vi "Get Parallel Sinks.vi"(8 "error in (no error)":errorcluster, 11 "Application Log in":refnum<class "Application Log.lvclass">) -> (0 "error out":errorcluster, 3 "Application Log out":refnum<class "Application Log.lvclass">, 5 "Parallel Sinks":bool)   [LabVIEW 2016, in "Stream Log.lvlib" / "Application Log.lvclass"]
doc: "--\nCopyright © 2017 Composed SystemsI All rights reserved.\n\nAuthor: Jon McBee <jon.mcbee@composed.io>\n\nThis library is provided \"AS IS\" ,WITHOUT WARRANTIES OR\nCONDITIONS OF ANY KIND, either express or implied.\n\nComposed Systems -- composed.io\n\nStream 0.0.1.1\nJon McBee - Composed Systems\nCopyright (c) 2017, Composed Systems"
uses:
  <userlib>/Composed Systems/Stream/Log/Application Log/Application Log.lvclass
  <userlib>/Composed Systems/Stream/Log/Application Log/Application Log.lvclass/Application Log.ctl
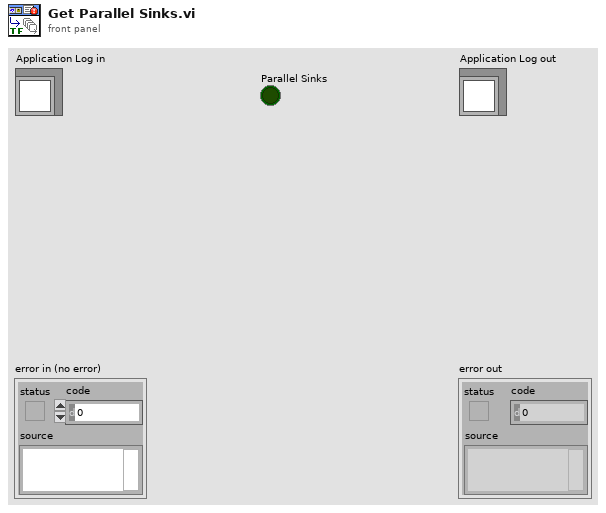
[diagram p1: front panel]
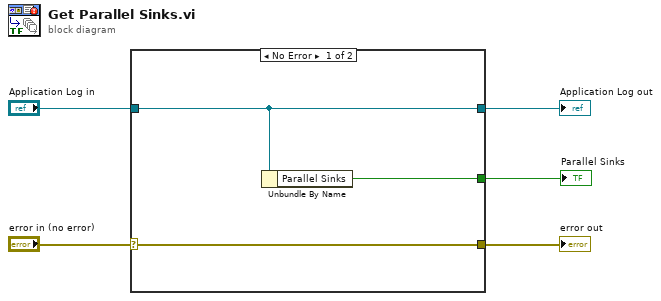
[diagram p0: block diagram]
diagram:
  n1 = case shown="No Error" "error in (no error)" {
    selector: "error in (no error)" -> [w8 w10]
    tunnel: [w8 w10] -> w4
    tunnel: [w7 w9] -> w2
    tunnel: "Application Log in" -> [w7 w9]
    tunnel: [w6 _] -> w1
    frame No Error {
      n2 = Unbundle By Name(w7) -> ("Parallel Sinks"=w6:bool)
    }
    frame Error {
    }
  }
  "error out" <- w4
  "Application Log out" <- w2
  "Parallel Sinks" <- w1
